vi "Motor Controller Command.vi"(8 "error in (no error)":errorcluster, 10 "Command":string, 11 "VISA resource name":refnum<visa-resource-name>) -> (0 "error out":errorcluster, 2 "Result":string, 3 "VISA resource name out":refnum<visa-resource-name>)   [LabVIEW 2011]
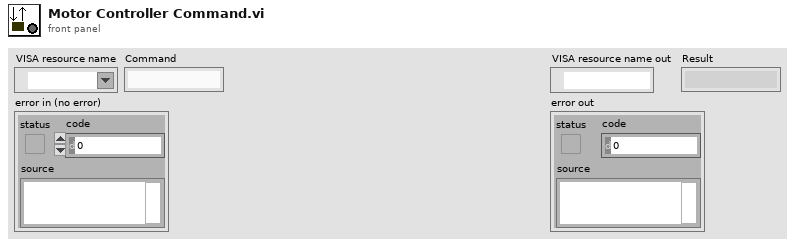
[diagram p1: front panel]
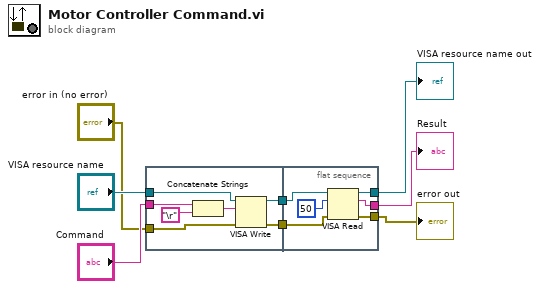
[diagram p0: block diagram]
diagram:
  n1 = flat-sequence {
    tunnel: [w15] -> w3
    tunnel: [w14] -> w2
    tunnel: "Command" -> [w11]
    tunnel: "VISA resource name" -> [w10]
    tunnel: "error in (no error)" -> [w9]
    tunnel: w3 -> [w21]
    tunnel: [w20] -> w4
    tunnel: w2 -> [w19]
    tunnel: [w18] -> w6
    tunnel: [w16] -> w5
    frame #0 {
      n2 = Concatenate Strings(w11, "\r") -> (w12:string)
      n3 = VISA Write(VISA resource name=w10, write buffer=w12, error in (no error)=w9) -> (VISA resource name out=w15:refnum<visa-resource-name>, error out=w14:errorcluster)  [unwired: 1 out]
    }
    frame #1 {
      n4 = VISA Read(VISA resource name=w21, byte count=u32 50, error in (no error)=w19) -> (VISA resource name out=w20:refnum<visa-resource-name>, read buffer=w16:string, error out=w18:errorcluster)  [unwired: 1 out]
    }
  }
  "VISA resource name out" <- w4
  "error out" <- w6
  "Result" <- w5
